vi "re_task.wakeup_lua.vi"(5 "LuaVIEW reference":T1) -> (15 "error out":errorcluster)   [LabVIEW 2012]
doc: "Wakes up a task. This causes an ongoing sleep() call of the task to return. When the task is otherwise occupied, its next sleep() call will drop through immediately. This function can be used to notify a task of some custom event.\nParameters:\nstr:task_identifier"
uses:
  typedefs/t_LuaVIEW Reference.ctl
  typedefs/t_LuaVIEW Task List Methods.ctl
  subvis/private/LuaVIEW Pull (string).vi
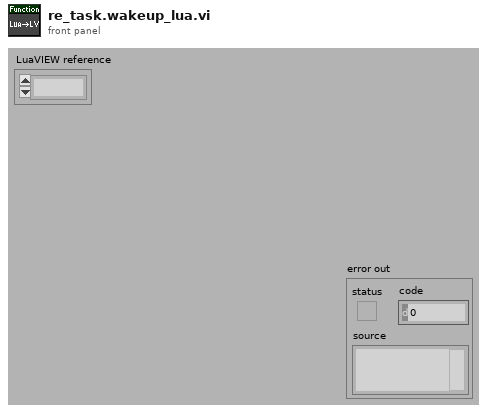
[diagram p1: front panel]
types:
  T1 = typedef "t_LuaVIEW Reference.ctl" = refnum<k1>
  T2 = typedef "t_LuaVIEW Task List Methods.ctl" = enum16{"clear list", "add", "test", "remove", "get ref", "get task info", "get list", "get script info", "ongoing?", "resume", "pause", "stop", "confirm", "message"}
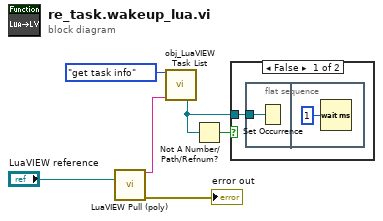
[diagram p0: block diagram]
diagram:
  n1 = call-poly "LuaVIEW Pull (poly).vi"("LuaVIEW reference in"="LuaVIEW reference") -> ("string"=w5:string, "error out"=→"error out":errorcluster)  [unwired: 12 in, 1 out]
  n2 = call "obj_LuaVIEW Task List.vi"("method"=t_LuaVIEW_Task_List_Methods."get task info", "task identifier"=w5) -> ("wakeup occurrence"=w1:refnum<k4>)  [unwired: 8 in, 5 out]
  n3 = Not A Number/Path/Refnum?(number/path/refnum=w1) -> (NaN/Path/Refnum?=w2:bool)
  n4 = case shown="False" w2 {
    tunnel: w1 -> [w7 _]
    frame False {
      n5 = flat-sequence {
        tunnel: w7 -> [w8]
        frame #0 {
          n6 = Set Occurrence(w8) -> ()
        }
        frame #1 {
          n7 = Wait (ms)(milliseconds to wait=u32 1) -> ()  [unwired: 1 out]
        }
      }
    }
    frame True {
    }
  }
